vi "Construct Rx.vi"(7 "error in (no error)":errorcluster, 9 "hardware channels":T1[](array[typedef]) {"channel settings"."Cluster"."DefaultCronoMode" items=["FDX_RX_DEFAULT_ENA_CNT", "FDX_RX_DEFAULT_MON_ENA_ALL", "FDX_RX_DEFAULT_MON_ENA_GOOD"]}, 10 "Custom Device Ref In":T4=18446744073709551615 format="%.0x") -> (0 "error out":errorcluster, 2 "Rx Execution Unit out":refnum<class "Rx Execution Unit.lvclass">, 3 "Custom Device Ref Out":T4=18446744073709551615 format="%.0x")   [LabVIEW 2020, in "afdx_custom_device Engine.lvlib" / "Implementation.lvlib" / "Rx Execution Unit.lvclass"]
uses:
  Rx Execution Unit.lvclass
  Execution Unit/Execution Unit.lvclass
  Execution Unit Factory/Execution Unit Factory.lvclass
  C:/repos/niveristand-aim-afdx-custom-device/Source/Custom Device Support/Engine/Implementation/Execution Unit/Execution Unit.lvclass
  C:/repos/niveristand-aim-afdx-custom-device/Source/Custom Device Support/Engine/Interfaces/Execution Unit/Execution Unit.lvclass
  C:/repos/niveristand-aim-afdx-custom-device/Source/Custom Device Support/Engine/Implementation/Rx Execution Unit/Rx Execution Unit.lvclass
  <vilib>/NI VeriStand/Custom Device API/Custom Device Item Ref.ctl
  <vilib>/NI VeriStand/Custom Device API/Custom Device API.lvlib
  AIM LabVIEW src/src/_controls/session_monitor_config.ctl
  AIM LabVIEW src/src/AIM664LV.lvlib
  channel_settings_rx.ctl
  hardware_channels_rx.ctl
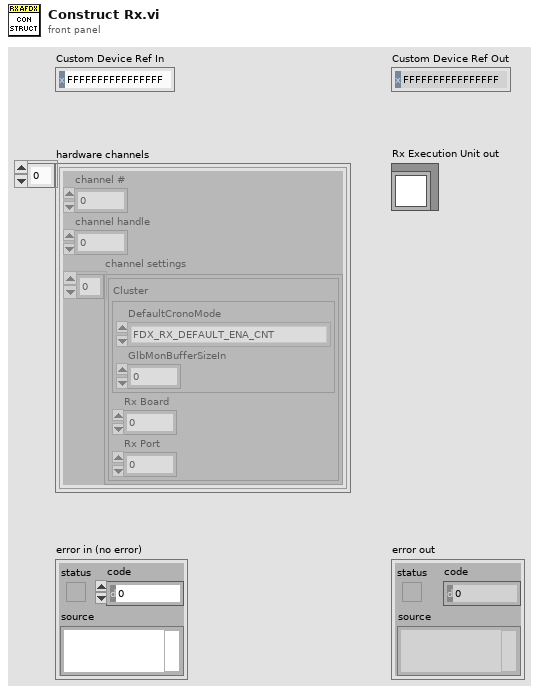
[diagram p1: front panel]
types:
  T1 = typedef "hardware_channels_rx.ctl" = cluster{"channel #":u16, "channel handle":u64, "channel settings":T2[]}
  T2 = typedef "channel_settings_rx.ctl" = cluster{"Cluster":T3, "Rx Board":dbl, "Rx Port":dbl}
  T3 = typedef "AIM664LV.lvlib/session_monitor_config.ctl" = cluster{"DefaultCronoMode":u32, "GlbMonBufferSizeIn":u32}
  T4 = typedef "Custom Device API.lvlib/Custom Device Item Ref.ctl" = u64
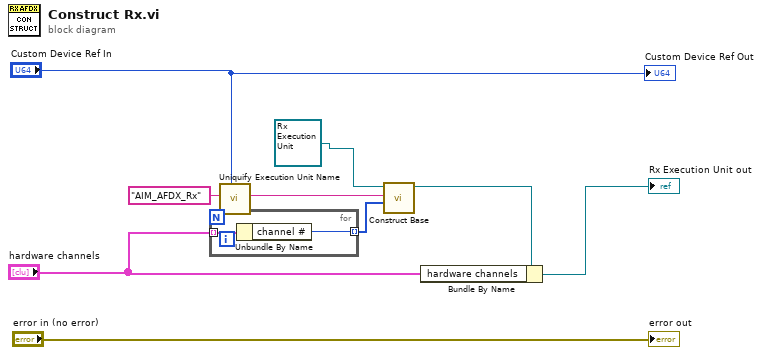
[diagram p0: block diagram]
diagram:
  n1 = for {
    tunnel: "hardware channels" -> [w11] mode=indexing
    tunnel: [w10] -> w4 mode=indexing
    n2 = Unbundle By Name(w11) -> ("channel #"=w10:u16)
  }
  n3 = call "Uniquify Execution Unit Name.vi"("custom device ref"="Custom Device Ref In", "execution unit name"="AIM_AFDX_Rx") -> ("execution unit name out"=w7:string)  [unwired: 9 in]
  n4 = call "Construct Base.vi"("Execution Unit Implementation (default object)"=refnum<class "Rx Execution Unit.lvclass"> refnum ("Communication Bus Template Interfaces:Implementation.lvlib:Rx Execution Unit.lvclass"), "identifier"=w7, "channels"=w4) -> ("Execution Unit Out"=w3:refnum<class "Rx Execution Unit.lvclass">)  [unwired: 6 in, 1 out]
  n5 = Bundle By Name(cluster=w3, "hardware channels"="hardware channels") -> (→"Rx Execution Unit out":refnum<class "Rx Execution Unit.lvclass">)
  "error out" <- "error in (no error)"
  "Custom Device Ref Out" <- "Custom Device Ref In"
